vi "Setup Motors.vi"   [LabVIEW 2014]
uses:
  <vilib>/Rock Robotics/SystemInterfaces/DIO/FPGA_DIOPWMChannel.ctl
  <vilib>/Rock Robotics/SystemInterfaces/Typedef/FPGA_TypedefDigitalModule.ctl
  <vilib>/Rock Robotics/WPI/Joystick/WPI_JoystickDeviceEnum.ctl
  <vilib>/Rock Robotics/SystemInterfaces/AI/FPGA_AIChannel.ctl
  <vilib>/Rock Robotics/SystemInterfaces/Typedef/FPGA_TypedefAnalogModule.ctl
  <vilib>/Rock Robotics/WPI/SafetyOutput/WPI_SafetyOutputConfigMenu.ctl
  <vilib>/Rock Robotics/WPI/Solenoid/WPI_SolenoidChannel.ctl
  <vilib>/Rock Robotics/SystemInterfaces/AI/FPGA_AIGyroChannel.ctl
  <vilib>/Rock Robotics/SystemInterfaces/Typedef/FPGA_TypedefAnalogModuleForGyro.ctl
  <vilib>/Rock Robotics/SystemInterfaces/DIO/FPGA_DIOChannel.ctl
  NavX Code/navX-MXP Library/COMMON/TypeDefs/Value TypeDefs/navX Interface Protocol.ctl
  <vilib>/Rock Robotics/SystemInterfaces/spilib/spi_bus.ctl
  <vilib>/Rock Robotics/SystemInterfaces/i2clib/i2c_bus.ctl
  NavX Code/navX-MXP Library/COMMON/TypeDefs/Value TypeDefs/navX Update Rate.ctl
  <vilib>/Rock Robotics/WPI/MotorControl/WPI_MotorControlOpen Jaguar.vi
  <vilib>/Rock Robotics/WPI/MotorControl/WPI_MotorControlOpen Talon.vi
  <vilib>/Rock Robotics/WPI/Solenoid/WPI_SolenoidOpenSingle.vi
  <vilib>/Rock Robotics/WPI/Switch/WPI_SwitchOpenLimit.vi
  <vilib>/Rock Robotics/WPI/Counter/WPI_CounterDigitalInputToDigitalSource.vi
  <vilib>/Rock Robotics/WPI/Counter/WPI_CounterOpen UpDown Mode.vi
  Global Variables.vi
  NavX Code/navX-MXP Library/navX-MXP IMU.lvlib
types:
  T1 = typedef "FPGA_DIOChannel.ctl" = enum8{"DIO 0", "DIO 1", "DIO 2", "DIO 3", "DIO 4", "DIO 5", "DIO 6", "DIO 7", "DIO 8", "DIO 9", "DIO MXP 0", "DIO MXP 1", "DIO MXP 2", "DIO MXP 3", "DIO MXP 4", "DIO MXP 5", "DIO MXP 6", "DIO MXP 7", "DIO MXP 8", "DIO MXP 9", "DIO MXP 10", "DIO MXP 11", "DIO MXP 12", "DIO MXP 13", "DIO MXP 14", "DIO MXP 15", "Invalid"}
  T2 = typedef "navX-MXP IMU.lvlib/navX Update Rate.ctl" = u8
  T3 = typedef "i2c_bus.ctl" = enum16{"I2C On-Board", "I2C MXP", "Invalid"}
  T4 = typedef "spi_bus.ctl" = enum16{"SPI On-Board, CS0", "SPI On-Board, CS1", "SPI On-Board, CS2", "SPI On-Board, CS3", "SPI MXP", "Invalid"}
  T5 = typedef "navX-MXP IMU.lvlib/navX Interface Protocol.ctl" = enum16{"SPI", "I2C"}
  T6 = typedef "WPI_SafetyOutputConfigMenu.ctl" = enum16{"Enable", "Disable"}
  T7 = typedef "FPGA_TypedefDigitalModule.ctl" = enum16{"Controller 1"}
  T8 = typedef "FPGA_TypedefAnalogModuleForGyro.ctl" = enum16{"Controller 1"}
  T9 = typedef "FPGA_AIGyroChannel.ctl" = enum8{"AI 0", "AI 1", "Invalid"}
  T10 = typedef "WPI_SolenoidChannel.ctl" = enum8{"Solenoid 0", "Solenoid 1", "Solenoid 2", "Solenoid 3", "Solenoid 4", "Solenoid 5", "Solenoid 6", "Solenoid 7", "Invalid"}
  T11 = typedef "FPGA_DIOPWMChannel.ctl" = enum8{"PWM 0", "PWM 1", "PWM 2", "PWM 3", "PWM 4", "PWM 5", "PWM 6", "PWM 7", "PWM 8", "PWM 9", "PWM MXP 0", "PWM MXP 1", "PWM MXP 2", "PWM MXP 3", "PWM MXP 4", "PWM MXP 5", "PWM MXP 6", "PWM MXP 7", "PWM MXP 8", "PWM MXP 9", "Invalid"}
  T12 = typedef "FPGA_AIChannel.ctl" = enum8{"AI 0", "AI 1", "AI 2", "AI 3", "AI MXP 0", "AI MXP 1", "AI MXP 2", "AI MXP 3", "Invalid"}
  T13 = typedef "FPGA_TypedefAnalogModule.ctl" = enum16{"Controller 1"}
  T14 = typedef "WPI_JoystickDeviceEnum.ctl" = enum16{"USB 0", "USB 1", "USB 2", "USB 3", "USB 4", "USB 5"}
  T15 = typedef "WPI_MotorControlDeviceRef.ctl" = cluster{"DeviceStatus":errorcluster, "Type":T16, "PWM":cluster{"Controller":T7, "PWM Channel":T11, "DeadBand":T17}, "CAN":cluster{"Device Number":u8, "Control Mode":T18, "Semaphore":T19, "Max Vout":dbl, "TalonSRX Control Mode":T20}, "Invert":bool, "TransformRef":T21, "InvTransformRef":T21}
  T16 = typedef "WPI_MotorControlType.ctl" = enum16{"PWM", "CAN", "CANTalonSRX"}
  T17 = typedef "WPI_PWMDeadband.ctl" = cluster{"Name":string, "maxPositivePwm":i32, "minPositivePwm":i32, "centerPwm":i32, "maxNegativePwm":i32, "minNegativePwm":i32, "angularRange":u16}
  T18 = typedef "WPI_CANJaguar_ControlMode.ctl" = enum8{"Percent VBus", "Current", "Speed", "Position", "Voltage"}
  T19 = typedef "Semaphore RefNum" = refnum<k1>
  T20 = typedef "WPI_CANTalonSRX_APIControlMode.ctl" = enum8{"Percent VBus", "Speed", "Position", "Slave", "Unchanged / Invalid"}
  T21 = typedef "WPI_PWMTransform_ConPane.ctl" = refnum<vi>
  T22 = typedef "WPI_SwitchDevRef.ctl" = cluster{"DevStatus":errorcluster, "DIO Channel":T1, "Controller":T7, "CntIndex":T23, "Normally Closed":bool}
  T23 = typedef "FPGA_CounterCtrSystemIndex.ctl" = enum8{"Ctr 0", "Ctr 1", "Ctr 2", "Ctr 3", "Ctr 4", "Ctr 5", "Ctr 6", "Ctr 7", "Invalid"}
  T24 = typedef "WPI_DigitalInputDevRef.ctl" = cluster{"DevStatus":errorcluster, "DIO Channel":T1, "Controller":T7}
  T25 = typedef "FPGA_CounterEncoderSourceConvertionLVSourceType.ctl" = cluster{"DevStatus":errorcluster, "AnalogTriggerMode?":bool, "DigitalMode":cluster{"Controller":T7, "DIO Channel":T26}, "AnalogTriggerMode":cluster{"AnalogTriggerIndex":T27, "OutputType":T28}}
  T26 = typedef "FPGA_DIODigitalSourceChannel.ctl" = enum8{"DIO 0", "DIO 1", "DIO 2", "DIO 3", "DIO 4", "DIO 5", "DIO 6", "DIO 7", "DIO 8", "DIO 9", "DIO MXP 0", "DIO MXP 1", "DIO MXP 2", "DIO MXP 3", "DIO MXP 4", "DIO MXP 5", "DIO MXP 6", "DIO MXP 7", "DIO MXP 8", "DIO MXP 9", "DIO MXP 10", "DIO MXP 11", "DIO MXP 12", "DIO MXP 13", "DIO MXP 14", "DIO MXP 15", "Disabled"}
  T27 = typedef "FPGA_AnalogTriggerIndex.ctl" = enum8{"Trig 0", "Trig 1", "Trig 2", "Trig 3", "Trig 4", "Trig 5", "Trig 6", "Trig 7", "Invalid"}
  T28 = typedef "FPGA_AnalogTriggerOutType.ctl" = enum16{"InWindow", "TriggerState", "Rising", "Falling"}
  T29 = typedef "WPI_EncoderDevRef.ctl" = cluster{"DevStatus":errorcluster, "EncoderIndex":T30, "CounterIndex":T23, "DistancePerCount":dbl, "Decoding Type":T31}
  T30 = typedef "FPGA_EncoderIdx.ctl" = enum8{"Enc 0", "Enc 1", "Enc 2", "Enc 3", "Enc 4", "Enc 5", "Enc 6", "Enc 7", "Invalid"}
  T31 = typedef "WPI_EncoderType.ctl" = enum16{"1x", "2x", "4x"}
  T32 = typedef "WPI_GyroDevRef.ctl" = cluster{"DevStatus":errorcluster, "Analog Module":T13, "Analog Channel":T12, "Offset":dbl, "Gain (VoltsPerDegree/Second)":dbl}
  T33 = typedef "WPI_SolenoidDevRef.ctl" = cluster{"DevStatus":errorcluster, "Pneumatics Control Module":u8, "Forward Solenoid Channel":T10, "Reverse Solenoid Channel":T10}
  T34 = typedef "WPI_AnalogChannelDevRef.ctl" = cluster{"DevStatus":errorcluster, "Controller":T13, "Analog Channel":T12}
  T35 = typedef "WPI_CounterDevRef.ctl" = cluster{"DevStatus":errorcluster, "CntIndex":T23}
  T36 = typedef "navX-MXP IMU.lvlib/navX Device TypeDef.ctl" = cluster{"navX Interface Protocol":T5, "navX Interface Protocol TypeDefs":cluster{"SPIDevRef":T37, "I2CDevRef":T38}, "navX System Information":cluster{"Board Information":T39, "Status":T40, "Offsets":T44}, "navX Common Information":cluster{"Update Rate (4Hz-60Hz)":T2, "refnum name":string, "error":errorcluster}}
  T37 = typedef "WPI_SPIDevRef.ctl" = cluster{"DevStatus":errorcluster, "Handle":i32, "Controller":T7, "SPI Bus":T4}
  T38 = typedef "WPI_I2CDevRef.ctl" = cluster{"DevStatus":errorcluster, "Controller":T7, "Device Address":u8, "Handle":i32, "I2C Bus":T3}
  T39 = typedef "navX-MXP IMU.lvlib/navX Board Information.ctl" = cluster{"WhoAmI (50 | 0x32)":u8, "Board Revision":u8, "Firmware Major Version":u8, "Firmware Minor Version":u8}
  T40 = typedef "navX-MXP IMU.lvlib/navX Status Data.ctl" = cluster{"Update Rate Hz":u8, "Accelerometer Full-Scale Range":u8, "Gyro Full-Scale Range":u16, "NAVX_OP_STATUS":T41, "NAVX_CAL_STATUS":T42, "NAVX_SELFTEST_STATUS":u8, "NAVX_SENSOR_STATUS":T43}
  T41 = typedef "navX-MXP IMU.lvlib/navX NAVX_OP_STATUS.ctl" = u8
  T42 = typedef "navX-MXP IMU.lvlib/navX NAVX_CAL_STATUS.ctl" = u8
  T43 = typedef "navX-MXP IMU.lvlib/navX NAVX_SENSOR_STATUS.ctl" = cluster{"MOVING":bool, "YAW_STABLE":bool, "MAG_DISTURBANCE":bool, "ALTITUDE_VALID":bool, "SEALEVEL_PRESS_SET":bool, "FUSED_HEADING_VALID":bool}
  T44 = typedef "navX-MXP IMU.lvlib/navX Offsets Data.ctl" = cluster{"Yaw":dbl, "Quat W":dbl, "Quat X":dbl, "Quat Y":dbl, "Quat Z":dbl}
  T45 = typedef "WPI_JoystickDevRef.ctl" = cluster{"Device":T14}
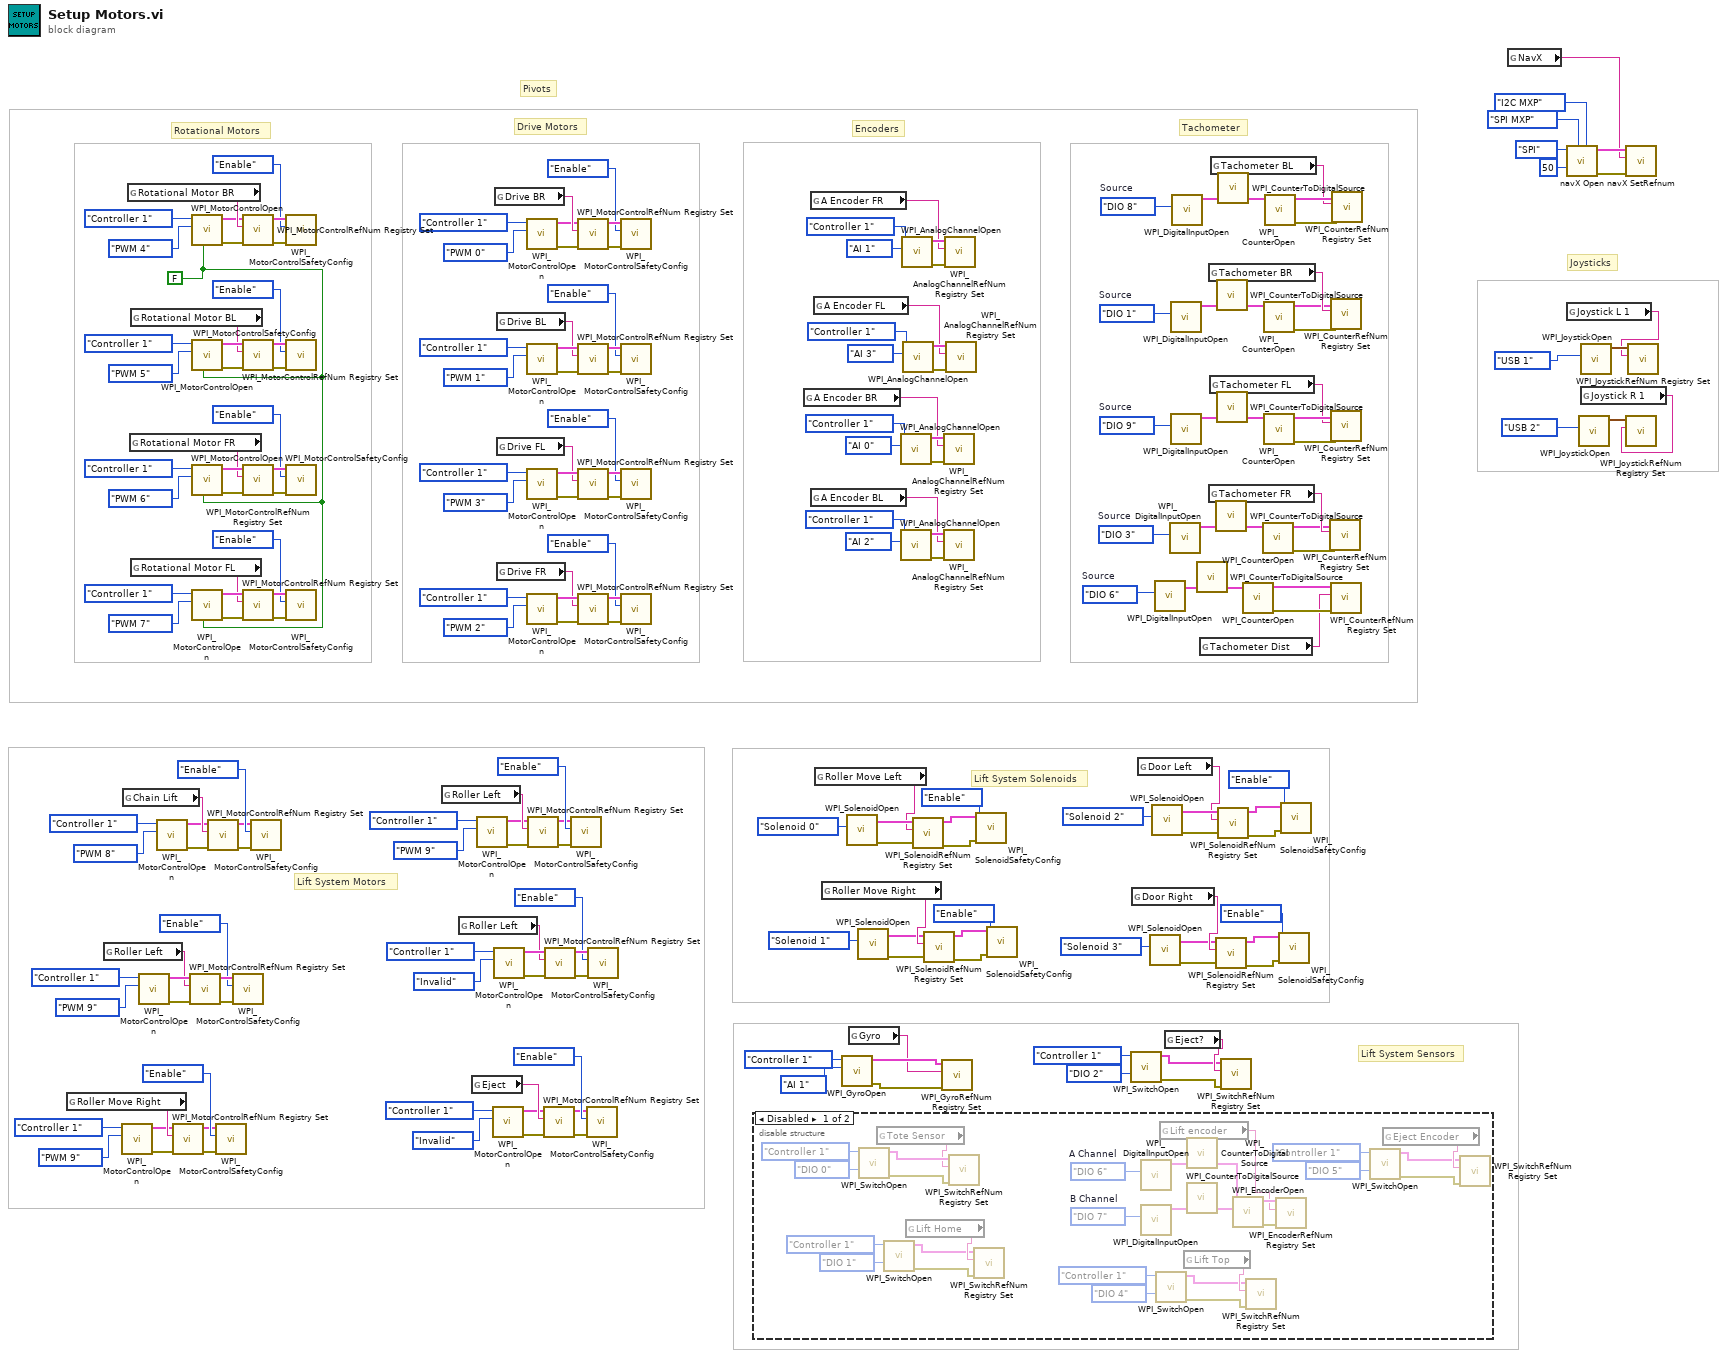
[diagram p0: block diagram]
diagram:
  w3 = FPGA_DIOChannel."DIO 6"  # Source
  w15 = FPGA_DIOChannel."DIO 3"  # Source
  w24 = FPGA_DIOChannel."DIO 9"  # Source
  w27 = FPGA_DIOChannel."DIO 1"  # Source
  w36 = FPGA_DIOChannel."DIO 8"  # Source
  w38 = FALSE ("Invert")
  # "Tachometer"
  # "Lift System Sensors"
  # "Lift System Solenoids"
  # "Lift System Motors"
  # "Encoders"
  # "Joysticks"
  # "Pivots"
  # "Rotational Motors"
  # "Drive Motors"
  n1 = global read "Global Variables.vi" "Roller Move Right"() -> (w107:string)
  n2 = global read "Global Variables.vi" "Roller Left"() -> (w110:string)
  n3 = call-poly <vilib>:"WPI_MotorControlOpen.vi"("PWM Channel"=FPGA_DIOPWMChannel."PWM 9", "Controller"=FPGA_TypedefDigitalModule."Controller 1") -> ("error out"=w102:errorcluster, "MotorControlDeviceRef"=w101:T15)  [unwired: 8 in]
  n4 = global read "Global Variables.vi" "Chain Lift"() -> (w123:string)
  n5 = global read "Global Variables.vi" "Rotational Motor BR"() -> (w177:string)
  n6 = global read "Global Variables.vi" "Rotational Motor FR"() -> (w151:string)
  n7 = global read "Global Variables.vi" "Rotational Motor BL"() -> (w152:string)
  n8 = global read "Global Variables.vi" "Rotational Motor FL"() -> (w150:string)
  n9 = call-poly <vilib>:"WPI_MotorControlOpen.vi"("PWM Channel"=FPGA_DIOPWMChannel."PWM 9", "Controller"=FPGA_TypedefDigitalModule."Controller 1") -> ("error out"=w115:errorcluster, "MotorControlDeviceRef"=w116:T15)  [unwired: 8 in]
  n10 = call-poly <vilib>:"WPI_MotorControlOpen.vi"("PWM Channel"=FPGA_DIOPWMChannel."PWM 8", "Controller"=FPGA_TypedefDigitalModule."Controller 1") -> ("error out"=w118:errorcluster, "MotorControlDeviceRef"=w117:T15)  [unwired: 8 in]
  n11 = call <vilib>:"WPI_MotorControlRefNum Registry Set.vi"("error in (no error)"=w102, "refnum name"=w107, "MotorControlDevRef"=w101) -> ("error out"=w104:errorcluster, "MotorControlDevRef"=w103:T15)  [unwired: 7 in]
  n12 = call <vilib>:"WPI_MotorControlRefNum Registry Set.vi"("error in (no error)"=w115, "refnum name"=w110, "MotorControlDevRef"=w116) -> ("error out"=w113:errorcluster, "MotorControlDevRef"=w114:T15)  [unwired: 7 in]
  n13 = call-poly <vilib>:"WPI_MotorControlOpen.vi"("Invert"=w38, "PWM Channel"=FPGA_DIOPWMChannel."PWM 4", "Controller"=FPGA_TypedefDigitalModule."Controller 1") -> ("error out"=w175:errorcluster, "MotorControlDeviceRef"=w176:T15)  [unwired: 7 in]
  n14 = call-poly <vilib>:"WPI_MotorControlOpen.vi"("Invert"=w38, "PWM Channel"=FPGA_DIOPWMChannel."PWM 5", "Controller"=FPGA_TypedefDigitalModule."Controller 1") -> ("error out"=w169:errorcluster, "MotorControlDeviceRef"=w170:T15)  [unwired: 7 in]
  n15 = call-poly <vilib>:"WPI_MotorControlOpen.vi"("Invert"=w38, "PWM Channel"=FPGA_DIOPWMChannel."PWM 6", "Controller"=FPGA_TypedefDigitalModule."Controller 1") -> ("error out"=w163:errorcluster, "MotorControlDeviceRef"=w164:T15)  [unwired: 7 in]
  n16 = call-poly <vilib>:"WPI_MotorControlOpen.vi"("Invert"=w38, "PWM Channel"=FPGA_DIOPWMChannel."PWM 7", "Controller"=FPGA_TypedefDigitalModule."Controller 1") -> ("error out"=w157:errorcluster, "MotorControlDeviceRef"=w158:T15)  [unwired: 7 in]
  n17 = call <vilib>:"WPI_MotorControlRefNum Registry Set.vi"("error in (no error)"=w118, "refnum name"=w123, "MotorControlDevRef"=w117) -> ("error out"=w120:errorcluster, "MotorControlDevRef"=w119:T15)  [unwired: 7 in]
  n18 = call <vilib>:"WPI_MotorControlSafetyConfig.vi"("error in (no error)"=w104, "mode"=WPI_SafetyOutputConfigMenu."Enable", "MotorControlDevRef"=w103) -> ()  [unwired: 7 in, 2 out]
  n19 = call <vilib>:"WPI_MotorControlSafetyConfig.vi"("error in (no error)"=w113, "mode"=WPI_SafetyOutputConfigMenu."Enable", "MotorControlDevRef"=w114) -> ()  [unwired: 7 in, 2 out]
  n20 = call <vilib>:"WPI_MotorControlRefNum Registry Set.vi"("error in (no error)"=w175, "refnum name"=w177, "MotorControlDevRef"=w176) -> ("error out"=w173:errorcluster, "MotorControlDevRef"=w174:T15)  [unwired: 7 in]
  n21 = call <vilib>:"WPI_MotorControlRefNum Registry Set.vi"("error in (no error)"=w169, "refnum name"=w152, "MotorControlDevRef"=w170) -> ("error out"=w167:errorcluster, "MotorControlDevRef"=w168:T15)  [unwired: 7 in]
  n22 = call <vilib>:"WPI_MotorControlRefNum Registry Set.vi"("error in (no error)"=w163, "refnum name"=w151, "MotorControlDevRef"=w164) -> ("error out"=w161:errorcluster, "MotorControlDevRef"=w162:T15)  [unwired: 7 in]
  n23 = call <vilib>:"WPI_MotorControlRefNum Registry Set.vi"("error in (no error)"=w157, "refnum name"=w150, "MotorControlDevRef"=w158) -> ("error out"=w155:errorcluster, "MotorControlDevRef"=w156:T15)  [unwired: 7 in]
  n24 = call <vilib>:"WPI_MotorControlSafetyConfig.vi"("error in (no error)"=w120, "mode"=WPI_SafetyOutputConfigMenu."Enable", "MotorControlDevRef"=w119) -> ()  [unwired: 7 in, 2 out]
  n25 = call <vilib>:"WPI_MotorControlSafetyConfig.vi"("error in (no error)"=w173, "mode"=WPI_SafetyOutputConfigMenu."Enable", "MotorControlDevRef"=w174) -> ()  [unwired: 7 in, 2 out]
  n26 = call <vilib>:"WPI_MotorControlSafetyConfig.vi"("error in (no error)"=w167, "mode"=WPI_SafetyOutputConfigMenu."Enable", "MotorControlDevRef"=w168) -> ()  [unwired: 7 in, 2 out]
  n27 = call <vilib>:"WPI_MotorControlSafetyConfig.vi"("error in (no error)"=w161, "mode"=WPI_SafetyOutputConfigMenu."Enable", "MotorControlDevRef"=w162) -> ()  [unwired: 7 in, 2 out]
  n28 = call <vilib>:"WPI_MotorControlSafetyConfig.vi"("error in (no error)"=w155, "mode"=WPI_SafetyOutputConfigMenu."Enable", "MotorControlDevRef"=w156) -> ()  [unwired: 7 in, 2 out]
  n29 = global read "Global Variables.vi" "Roller Left"() -> (w99:string)
  n30 = global read "Global Variables.vi" "Roller Left"() -> (w86:string)
  n31 = global read "Global Variables.vi" "Eject"() -> (w83:string)
  n32 = call-poly <vilib>:"WPI_MotorControlOpen.vi"("PWM Channel"=FPGA_DIOPWMChannel."PWM 9", "Controller"=FPGA_TypedefDigitalModule."Controller 1") -> ("error out"=w94:errorcluster, "MotorControlDeviceRef"=w93:T15)  [unwired: 8 in]
  n33 = call-poly <vilib>:"WPI_MotorControlOpen.vi"("PWM Channel"=FPGA_DIOPWMChannel."Invalid", "Controller"=FPGA_TypedefDigitalModule."Controller 1") -> ("error out"=w78:errorcluster, "MotorControlDeviceRef"=w77:T15)  [unwired: 8 in]
  n34 = call-poly <vilib>:"WPI_MotorControlOpen.vi"("PWM Channel"=FPGA_DIOPWMChannel."Invalid", "Controller"=FPGA_TypedefDigitalModule."Controller 1") -> ("error out"=w91:errorcluster, "MotorControlDeviceRef"=w92:T15)  [unwired: 8 in]
  n35 = global read "Global Variables.vi" "Drive BR"() -> (w214:string)
  n36 = global read "Global Variables.vi" "Drive BL"() -> (w189:string)
  n37 = global read "Global Variables.vi" "Drive FL"() -> (w188:string)
  n38 = global read "Global Variables.vi" "Drive FR"() -> (w187:string)
  n39 = call-poly <vilib>:"WPI_MotorControlOpen.vi"("PWM Channel"=FPGA_DIOPWMChannel."PWM 0", "Controller"=FPGA_TypedefDigitalModule."Controller 1") -> ("error out"=w212:errorcluster, "MotorControlDeviceRef"=w213:T15)  [unwired: 8 in]
  n40 = call-poly <vilib>:"WPI_MotorControlOpen.vi"("PWM Channel"=FPGA_DIOPWMChannel."PWM 1", "Controller"=FPGA_TypedefDigitalModule."Controller 1") -> ("error out"=w206:errorcluster, "MotorControlDeviceRef"=w207:T15)  [unwired: 8 in]
  n41 = call-poly <vilib>:"WPI_MotorControlOpen.vi"("PWM Channel"=FPGA_DIOPWMChannel."PWM 3", "Controller"=FPGA_TypedefDigitalModule."Controller 1") -> ("error out"=w200:errorcluster, "MotorControlDeviceRef"=w201:T15)  [unwired: 8 in]
  n42 = call-poly <vilib>:"WPI_MotorControlOpen.vi"("PWM Channel"=FPGA_DIOPWMChannel."PWM 2", "Controller"=FPGA_TypedefDigitalModule."Controller 1") -> ("error out"=w194:errorcluster, "MotorControlDeviceRef"=w195:T15)  [unwired: 8 in]
  n43 = call <vilib>:"WPI_MotorControlRefNum Registry Set.vi"("error in (no error)"=w94, "refnum name"=w99, "MotorControlDevRef"=w93) -> ("error out"=w96:errorcluster, "MotorControlDevRef"=w95:T15)  [unwired: 7 in]
  n44 = call <vilib>:"WPI_MotorControlRefNum Registry Set.vi"("error in (no error)"=w78, "refnum name"=w83, "MotorControlDevRef"=w77) -> ("error out"=w80:errorcluster, "MotorControlDevRef"=w79:T15)  [unwired: 7 in]
  n45 = call <vilib>:"WPI_MotorControlRefNum Registry Set.vi"("error in (no error)"=w91, "refnum name"=w86, "MotorControlDevRef"=w92) -> ("error out"=w89:errorcluster, "MotorControlDevRef"=w90:T15)  [unwired: 7 in]
  n46 = call <vilib>:"WPI_MotorControlSafetyConfig.vi"("error in (no error)"=w96, "mode"=WPI_SafetyOutputConfigMenu."Enable", "MotorControlDevRef"=w95) -> ()  [unwired: 7 in, 2 out]
  n47 = call <vilib>:"WPI_MotorControlRefNum Registry Set.vi"("error in (no error)"=w212, "refnum name"=w214, "MotorControlDevRef"=w213) -> ("error out"=w210:errorcluster, "MotorControlDevRef"=w211:T15)  [unwired: 7 in]
  n48 = call <vilib>:"WPI_MotorControlRefNum Registry Set.vi"("error in (no error)"=w206, "refnum name"=w189, "MotorControlDevRef"=w207) -> ("error out"=w204:errorcluster, "MotorControlDevRef"=w205:T15)  [unwired: 7 in]
  n49 = call <vilib>:"WPI_MotorControlRefNum Registry Set.vi"("error in (no error)"=w200, "refnum name"=w188, "MotorControlDevRef"=w201) -> ("error out"=w198:errorcluster, "MotorControlDevRef"=w199:T15)  [unwired: 7 in]
  n50 = call <vilib>:"WPI_MotorControlRefNum Registry Set.vi"("error in (no error)"=w194, "refnum name"=w187, "MotorControlDevRef"=w195) -> ("error out"=w192:errorcluster, "MotorControlDevRef"=w193:T15)  [unwired: 7 in]
  n51 = call <vilib>:"WPI_MotorControlSafetyConfig.vi"("error in (no error)"=w80, "mode"=WPI_SafetyOutputConfigMenu."Enable", "MotorControlDevRef"=w79) -> ()  [unwired: 7 in, 2 out]
  n52 = call <vilib>:"WPI_MotorControlSafetyConfig.vi"("error in (no error)"=w89, "mode"=WPI_SafetyOutputConfigMenu."Enable", "MotorControlDevRef"=w90) -> ()  [unwired: 7 in, 2 out]
  n53 = call <vilib>:"WPI_MotorControlSafetyConfig.vi"("error in (no error)"=w210, "mode"=WPI_SafetyOutputConfigMenu."Enable", "MotorControlDevRef"=w211) -> ()  [unwired: 7 in, 2 out]
  n54 = call <vilib>:"WPI_MotorControlSafetyConfig.vi"("error in (no error)"=w204, "mode"=WPI_SafetyOutputConfigMenu."Enable", "MotorControlDevRef"=w205) -> ()  [unwired: 7 in, 2 out]
  n55 = call <vilib>:"WPI_MotorControlSafetyConfig.vi"("error in (no error)"=w198, "mode"=WPI_SafetyOutputConfigMenu."Enable", "MotorControlDevRef"=w199) -> ()  [unwired: 7 in, 2 out]
  n56 = call <vilib>:"WPI_MotorControlSafetyConfig.vi"("error in (no error)"=w192, "mode"=WPI_SafetyOutputConfigMenu."Enable", "MotorControlDevRef"=w193) -> ()  [unwired: 7 in, 2 out]
  n57 = disable-structure shown="Disabled" {
    frame Disabled {
      w223 = FPGA_DIOChannel."DIO 7"  # B Channel
      w222 = FPGA_DIOChannel."DIO 6"  # A Channel
      n58 = call-poly <vilib>:"WPI_SwitchOpen.vi"("DIO Channel"=FPGA_DIOChannel."DIO 0", "Controller"=FPGA_TypedefDigitalModule."Controller 1") -> ("error out"=w242:errorcluster, "SwitchDevRef"=w243:T22)  [unwired: 8 in]
      n59 = global read "Global Variables.vi" "Tote Sensor"() -> (w239:string)
      n60 = call-poly <vilib>:"WPI_SwitchOpen.vi"("DIO Channel"=FPGA_DIOChannel."DIO 1", "Controller"=FPGA_TypedefDigitalModule."Controller 1") -> ("error out"=w235:errorcluster, "SwitchDevRef"=w234:T22)  [unwired: 8 in]
      n61 = global read "Global Variables.vi" "Lift Home"() -> (w238:string)
      n62 = call <vilib>:"WPI_SwitchRefNum Registry Set.vi"("error in (no error)"=w242, "refnum name"=w239, "SwitchDevRef"=w243) -> ()  [unwired: 7 in, 2 out]
      n63 = call <vilib>:"WPI_SwitchRefNum Registry Set.vi"("error in (no error)"=w235, "refnum name"=w238, "SwitchDevRef"=w234) -> ()  [unwired: 7 in, 2 out]
      n64 = call <vilib>:"WPI_DigitalInputOpen.vi"("DIO Channel"=w222) -> ("DigitalInputDevRef"=w219:T24)  [unwired: 2 in, 8 out]
      n65 = call <vilib>:"WPI_DigitalInputOpen.vi"("DIO Channel"=w223) -> ("DigitalInputDevRef"=w220:T24)  [unwired: 2 in, 8 out]
      n66 = call-poly <vilib>:"WPI_SwitchOpen.vi"("DIO Channel"=FPGA_DIOChannel."DIO 4", "Controller"=FPGA_TypedefDigitalModule."Controller 1") -> ("error out"=w230:errorcluster, "SwitchDevRef"=w229:T22)  [unwired: 8 in]
      n67 = global read "Global Variables.vi" "Lift encoder"() -> (w215:string)
      n68 = global read "Global Variables.vi" "Lift Top"() -> (w233:string)
      n69 = call-poly <vilib>:"WPI_CounterToDigitalSource.vi"("DigitalInputDevRef"=w219) -> ("Digital Source"=w218:T25)  [unwired: 6 out]
      n70 = call-poly <vilib>:"WPI_CounterToDigitalSource.vi"("DigitalInputDevRef"=w220) -> ("Digital Source"=w221:T25)  [unwired: 6 out]
      n71 = call <vilib>:"WPI_EncoderOpen.vi"("BSource"=w221, "ASource"=w218) -> ("error out"=w217:errorcluster, "EncoderDevRef"=w216:T29)  [unwired: 6 in, 2 out]
      n72 = call <vilib>:"WPI_SwitchRefNum Registry Set.vi"("error in (no error)"=w230, "refnum name"=w233, "SwitchDevRef"=w229) -> ()  [unwired: 7 in, 2 out]
      n73 = call <vilib>:"WPI_EncoderRefNum Registry Set.vi"("error in (no error)"=w217, "refnum name"=w215, "EncoderDevRef"=w216) -> ()  [unwired: 7 in, 2 out]
      n74 = call-poly <vilib>:"WPI_SwitchOpen.vi"("DIO Channel"=FPGA_DIOChannel."DIO 5", "Controller"=FPGA_TypedefDigitalModule."Controller 1") -> ("error out"=w225:errorcluster, "SwitchDevRef"=w224:T22)  [unwired: 8 in]
      n75 = global read "Global Variables.vi" "Eject Encoder"() -> (w228:string)
      n76 = call <vilib>:"WPI_SwitchRefNum Registry Set.vi"("error in (no error)"=w225, "refnum name"=w228, "SwitchDevRef"=w224) -> ()  [unwired: 7 in, 2 out]
    }
    frame Enabled {
    }
  }
  n77 = global read "Global Variables.vi" "A Encoder BR"() -> (w126:string)
  n78 = global read "Global Variables.vi" "A Encoder FR"() -> (w128:string)
  n79 = global read "Global Variables.vi" "A Encoder BL"() -> (w127:string)
  n80 = global read "Global Variables.vi" "A Encoder FL"() -> (w125:string)
  n81 = global read "Global Variables.vi" "Roller Move Left"() -> (w71:string)
  n82 = global read "Global Variables.vi" "Roller Move Right"() -> (w70:string)
  n83 = call <vilib>:"WPI_GyroOpen.vi"("Analog Channel"=FPGA_AIGyroChannel."AI 1", "Controller"=FPGA_TypedefAnalogModuleForGyro."Controller 1") -> ("error out"=w51:errorcluster, "GyroDevRef"=w52:T32)  [unwired: 7 in, 1 out]
  n84 = call-poly <vilib>:"WPI_SolenoidOpen.vi"("Solenoid Channel"=WPI_SolenoidChannel."Solenoid 0") -> ("error out"=w73:errorcluster, "SolenoidDevRef"=w74:T33)  [unwired: 9 in]
  n85 = global read "Global Variables.vi" "Gyro"() -> (w48:string)
  n86 = call-poly <vilib>:"WPI_SolenoidOpen.vi"("Solenoid Channel"=WPI_SolenoidChannel."Solenoid 1") -> ("error out"=w68:errorcluster, "SolenoidDevRef"=w67:T33)  [unwired: 9 in]
  n87 = call <vilib>:"WPI_AnalogChannelOpen.vi"("Analog Channel"=FPGA_AIChannel."AI 0", "Controller"=FPGA_TypedefAnalogModule."Controller 1") -> ("error out"=w135:errorcluster, "AIDeviceRef"=w136:T34)  [unwired: 8 in]
  n88 = call <vilib>:"WPI_AnalogChannelOpen.vi"("Analog Channel"=FPGA_AIChannel."AI 2", "Controller"=FPGA_TypedefAnalogModule."Controller 1") -> ("error out"=w131:errorcluster, "AIDeviceRef"=w132:T34)  [unwired: 8 in]
  n89 = call <vilib>:"WPI_AnalogChannelOpen.vi"("Analog Channel"=FPGA_AIChannel."AI 1", "Controller"=FPGA_TypedefAnalogModule."Controller 1") -> ("error out"=w143:errorcluster, "AIDeviceRef"=w144:T34)  [unwired: 8 in]
  n90 = call <vilib>:"WPI_AnalogChannelOpen.vi"("Analog Channel"=FPGA_AIChannel."AI 3", "Controller"=FPGA_TypedefAnalogModule."Controller 1") -> ("error out"=w139:errorcluster, "AIDeviceRef"=w140:T34)  [unwired: 8 in]
  n91 = call <vilib>:"WPI_SolenoidRefNum Registry Set.vi"("error in (no error)"=w73, "refnum name"=w71, "SolenoidDevRef"=w74) -> ("error out"=w75:errorcluster, "SolenoidDevRef"=w76:T33)  [unwired: 7 in]
  n92 = call <vilib>:"WPI_SolenoidRefNum Registry Set.vi"("error in (no error)"=w68, "refnum name"=w70, "SolenoidDevRef"=w67) -> ("error out"=w66:errorcluster, "SolenoidDevRef"=w65:T33)  [unwired: 7 in]
  n93 = call <vilib>:"WPI_GyroRefNum Registry Set.vi"("error in (no error)"=w51, "refnum name"=w48, "GyroDevRef"=w52) -> ()  [unwired: 7 in, 2 out]
  n94 = call <vilib>:"WPI_AnalogChannelRefNum Registry Set.vi"("error in (no error)"=w135, "refnum name"=w126, "AIDeviceRef"=w136) -> ()  [unwired: 7 in, 2 out]
  n95 = call <vilib>:"WPI_AnalogChannelRefNum Registry Set.vi"("error in (no error)"=w131, "refnum name"=w127, "AIDeviceRef"=w132) -> ()  [unwired: 7 in, 2 out]
  n96 = call <vilib>:"WPI_AnalogChannelRefNum Registry Set.vi"("error in (no error)"=w143, "refnum name"=w128, "AIDeviceRef"=w144) -> ()  [unwired: 7 in, 2 out]
  n97 = call <vilib>:"WPI_AnalogChannelRefNum Registry Set.vi"("error in (no error)"=w139, "refnum name"=w125, "AIDeviceRef"=w140) -> ()  [unwired: 7 in, 2 out]
  n98 = call <vilib>:"WPI_SolenoidSafetyConfig.vi"("error in (no error)"=w75, "mode"=WPI_SafetyOutputConfigMenu."Enable", "SolenoidDevRef"=w76) -> ()  [unwired: 7 in, 2 out]
  n99 = call <vilib>:"WPI_SolenoidSafetyConfig.vi"("error in (no error)"=w66, "mode"=WPI_SafetyOutputConfigMenu."Enable", "SolenoidDevRef"=w65) -> ()  [unwired: 7 in, 2 out]
  n100 = call-poly <vilib>:"WPI_SwitchOpen.vi"("DIO Channel"=FPGA_DIOChannel."DIO 2", "Controller"=FPGA_TypedefDigitalModule."Controller 1") -> ("error out"=w44:errorcluster, "SwitchDevRef"=w43:T22)  [unwired: 8 in]
  n101 = global read "Global Variables.vi" "Door Right"() -> (w58:string)
  n102 = global read "Global Variables.vi" "Door Left"() -> (w59:string)
  n103 = call-poly <vilib>:"WPI_SolenoidOpen.vi"("Solenoid Channel"=WPI_SolenoidChannel."Solenoid 3") -> ("error out"=w56:errorcluster, "SolenoidDevRef"=w55:T33)  [unwired: 9 in]
  n104 = call-poly <vilib>:"WPI_SolenoidOpen.vi"("Solenoid Channel"=WPI_SolenoidChannel."Solenoid 2") -> ("error out"=w61:errorcluster, "SolenoidDevRef"=w62:T33)  [unwired: 9 in]
  n105 = call <vilib>:"WPI_DigitalInputOpen.vi"("DIO Channel"=w3) -> ("DigitalInputDevRef"=w6:T24)  [unwired: 2 in, 8 out]
  n106 = global read "Global Variables.vi" "Eject?"() -> (w47:string)
  n107 = call <vilib>:"WPI_DigitalInputOpen.vi"("DIO Channel"=w15) -> ("DigitalInputDevRef"=w16:T24)  [unwired: 2 in, 8 out]
  n108 = call <vilib>:"WPI_DigitalInputOpen.vi"("DIO Channel"=w27) -> ("DigitalInputDevRef"=w28:T24)  [unwired: 2 in, 8 out]
  n109 = call <vilib>:"WPI_DigitalInputOpen.vi"("DIO Channel"=w24) -> ("DigitalInputDevRef"=w23:T24)  [unwired: 2 in, 8 out]
  n110 = call <vilib>:"WPI_DigitalInputOpen.vi"("DIO Channel"=w36) -> ("DigitalInputDevRef"=w35:T24)  [unwired: 2 in, 8 out]
  n111 = call-poly <vilib>:"WPI_CounterToDigitalSource.vi"("DigitalInputDevRef"=w6) -> ("Digital Source"=w5:T25)  [unwired: 6 out]
  n112 = global read "Global Variables.vi" "Tachometer Dist"() -> (w1:string)
  n113 = global read "Global Variables.vi" "Tachometer BR"() -> (w31:string)
  n114 = global read "Global Variables.vi" "Tachometer FR"() -> (w19:string)
  n115 = global read "Global Variables.vi" "Tachometer FL"() -> (w20:string)
  n116 = global read "Global Variables.vi" "Tachometer BL"() -> (w32:string)
  n117 = call-poly <vilib>:"WPI_CounterToDigitalSource.vi"("DigitalInputDevRef"=w16) -> ("Digital Source"=w14:T25)  [unwired: 6 out]
  n118 = call <vilib>:"WPI_SolenoidRefNum Registry Set.vi"("error in (no error)"=w56, "refnum name"=w58, "SolenoidDevRef"=w55) -> ("error out"=w54:errorcluster, "SolenoidDevRef"=w53:T33)  [unwired: 7 in]
  n119 = call-poly <vilib>:"WPI_CounterToDigitalSource.vi"("DigitalInputDevRef"=w28) -> ("Digital Source"=w26:T25)  [unwired: 6 out]
  n120 = call-poly <vilib>:"WPI_CounterToDigitalSource.vi"("DigitalInputDevRef"=w23) -> ("Digital Source"=w25:T25)  [unwired: 6 out]
  n121 = call-poly <vilib>:"WPI_CounterToDigitalSource.vi"("DigitalInputDevRef"=w35) -> ("Digital Source"=w37:T25)  [unwired: 6 out]
  n122 = call <vilib>:"WPI_SolenoidRefNum Registry Set.vi"("error in (no error)"=w61, "refnum name"=w59, "SolenoidDevRef"=w62) -> ("error out"=w63:errorcluster, "SolenoidDevRef"=w64:T33)  [unwired: 7 in]
  n123 = call <vilib>:"WPI_SwitchRefNum Registry Set.vi"("error in (no error)"=w44, "refnum name"=w47, "SwitchDevRef"=w43) -> ()  [unwired: 7 in, 2 out]
  n124 = call-poly <vilib>:"WPI_CounterOpen.vi"("Up Source"=w5) -> ("error out"=w2:errorcluster, "CounterDevRef"=w4:T35)  [unwired: 6 in, 3 out]
  n125 = call-poly <vilib>:"WPI_CounterOpen.vi"("Up Source"=w14) -> ("error out"=w18:errorcluster, "CounterDevRef"=w17:T35)  [unwired: 6 in, 3 out]
  n126 = call-poly <vilib>:"WPI_CounterOpen.vi"("Up Source"=w26) -> ("error out"=w30:errorcluster, "CounterDevRef"=w29:T35)  [unwired: 6 in, 3 out]
  n127 = call-poly <vilib>:"WPI_CounterOpen.vi"("Up Source"=w25) -> ("error out"=w21:errorcluster, "CounterDevRef"=w22:T35)  [unwired: 6 in, 3 out]
  n128 = call-poly <vilib>:"WPI_CounterOpen.vi"("Up Source"=w37) -> ("error out"=w33:errorcluster, "CounterDevRef"=w34:T35)  [unwired: 6 in, 3 out]
  n129 = call <vilib>:"WPI_SolenoidSafetyConfig.vi"("error in (no error)"=w54, "mode"=WPI_SafetyOutputConfigMenu."Enable", "SolenoidDevRef"=w53) -> ()  [unwired: 7 in, 2 out]
  n130 = call <vilib>:"WPI_SolenoidSafetyConfig.vi"("error in (no error)"=w63, "mode"=WPI_SafetyOutputConfigMenu."Enable", "SolenoidDevRef"=w64) -> ()  [unwired: 7 in, 2 out]
  n131 = call <vilib>:"WPI_CounterRefNum Registry Set.vi"("error in (no error)"=w18, "refnum name"=w19, "CounterDevRef"=w17) -> ()  [unwired: 7 in, 2 out]
  n132 = call <vilib>:"WPI_CounterRefNum Registry Set.vi"("error in (no error)"=w30, "refnum name"=w31, "CounterDevRef"=w29) -> ()  [unwired: 7 in, 2 out]
  n133 = call <vilib>:"WPI_CounterRefNum Registry Set.vi"("error in (no error)"=w21, "refnum name"=w20, "CounterDevRef"=w22) -> ()  [unwired: 7 in, 2 out]
  n134 = call <vilib>:"WPI_CounterRefNum Registry Set.vi"("error in (no error)"=w2, "refnum name"=w1, "CounterDevRef"=w4) -> ()  [unwired: 7 in, 2 out]
  n135 = call <vilib>:"WPI_CounterRefNum Registry Set.vi"("error in (no error)"=w33, "refnum name"=w32, "CounterDevRef"=w34) -> ()  [unwired: 7 in, 2 out]
  n136 = global read "Global Variables.vi" "NavX"() -> (w7:string)
  n137 = call "navX Open.vi"("I2C Bus"=i2c_bus."I2C MXP", "SPI Bus"=spi_bus."SPI MXP", "Update Rate (4Hz-60Hz)"=T2 50, "navX Interface Protocol"=navX_Interface_Protocol."SPI") -> ("error out"=w9:errorcluster, "navX Device TypeDef"=w8:T36)  [unwired: 5 in, 1 out]
  n138 = global read "Global Variables.vi" "Joystick L 1"() -> (w181:string)
  n139 = call <vilib>:"WPI_JoystickOpen.vi"("JoystickDevice"=WPI_JoystickDeviceEnum."USB 2") -> ("JoystickDevRef"=w179:T45)  [unwired: 10 in]
  n140 = call <vilib>:"WPI_JoystickOpen.vi"("JoystickDevice"=WPI_JoystickDeviceEnum."USB 1") -> ("JoystickDevRef"=w182:T45)  [unwired: 10 in]
  n141 = global read "Global Variables.vi" "Joystick R 1"() -> (w178:string)
  n142 = call "navX SetRefnum.vi"("error in (no error)"=w9, "refnum name"=w7, "navX Device TypeDef"=w8) -> ()  [unwired: 7 in, 2 out]
  n143 = call <vilib>:"WPI_JoystickRefNum Registry Set.vi"("refnum name"=w178, "JoystickDevRef"=w179) -> ()  [unwired: 8 in, 2 out]
  n144 = call <vilib>:"WPI_JoystickRefNum Registry Set.vi"("refnum name"=w181, "JoystickDevRef"=w182) -> ()  [unwired: 8 in, 2 out]
